vi "Read Pattern from disk.vi"() -> ()   [LabVIEW 2011]
panel:
  out "Intensity Graph":u8[][](graph)
  out "output array":u8[][](array[numeric])
  out "error out":errorcluster
  in  "File Path Control":path=path "C:/Data/Antonio/software/LCOS/LCOS_CompleteLV/python/pattern_800x600_uint8_C_order.bin"
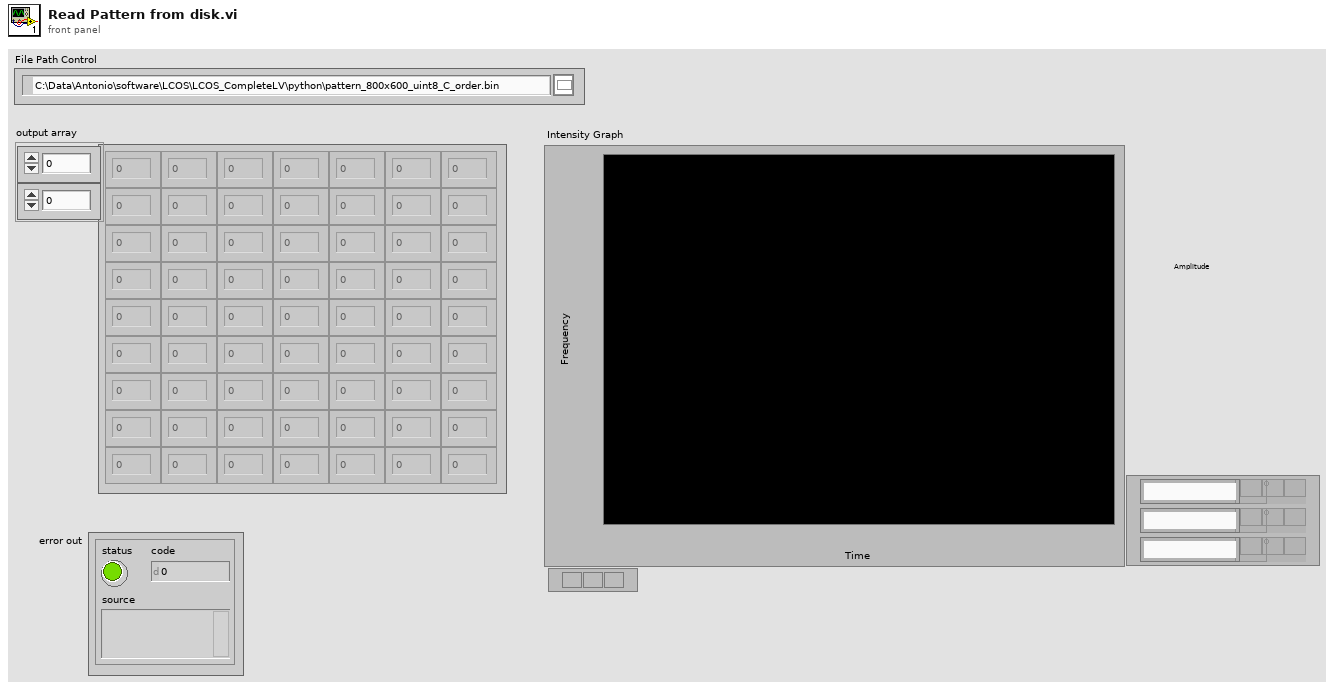
[diagram p1: front panel]
types:
  T1 = enum16{"big-endian, network order", "native, host order", "little-endian"}
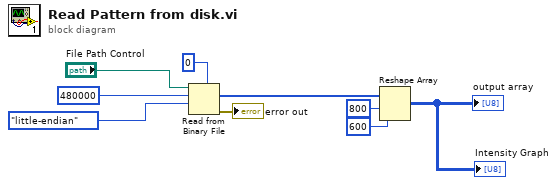
[diagram p0: block diagram]
diagram:
  n1 = Read from Binary File(5:u8 0, 9:T1."little-endian" ("byte order (0:big-endian, network order)"), 10:480000 ("count (1)"), 11:"File Path Control") -> (0:→"error out":errorcluster, 2:w4:u8[])  [unwired: 2 in, 2 out]
  n2 = Reshape Array(w4, 800 ("dimension size"), 600 ("dimension size")) -> (→"output array" →"Intensity Graph":u8[][])
